vi "SV Get Data Subset.vi"   [LabVIEW 2017]
doc: "Returns a portion of the waveform of the <B>start index</B> and <B>length</B> values. When you wire a waveform to this VI, the waveform automatically resizes to display <B>start index</B> inputs for the waveform."
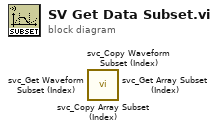
[diagram p0: block diagram]
diagram:
  n1 = call <vilib>:"svc_Copy Array Subset (Index).vi"() -> ()  [unwired: 7 in, 5 out]
  n2 = call <vilib>:"svc_Copy Waveform Subset (Index).vi"() -> ()  [unwired: 7 in, 5 out]
  n3 = call <vilib>:"svc_Get Waveform Subset (Index).vi"() -> ()  [unwired: 6 in, 6 out]
  n4 = call <vilib>:"svc_Get Array Subset (Index).vi"() -> ()  [unwired: 7 in, 5 out]
